vi "IrDA-Client.vi"() -> ()   [LabVIEW 2019]
doc: "Demonstrates how to open a connection to an IrDA server, read the data being sent, and display the data on a chart. This VI is designed to stop if the IrDA connection is terminated."
panel:
  in  "Server Closed":string="The server VI closed the connection."
  out "Waveform Graph":dbl[](graph)
  in  "Stop":bool
  # "Overview: Demonstrates the use of the IrDA functions to connect to an IrDA server VI and receive data.\nRequirements: IrDA-enabled computer\nInstructions:\n1. Ensure Simple IrDA - Server.vi is already running.\n2. Run the VI.\n3. Click Stop to stop the VI. Note that if you stop the server VI, this VI will stop automatically."
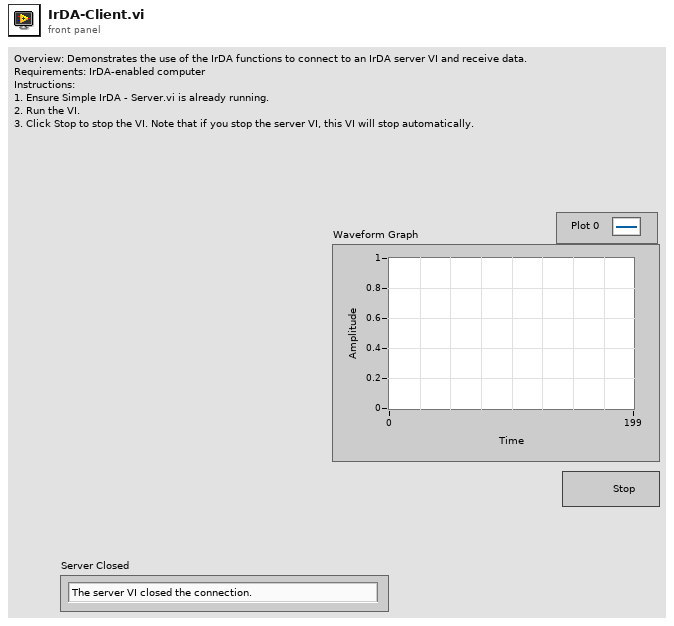
[diagram p1: front panel]
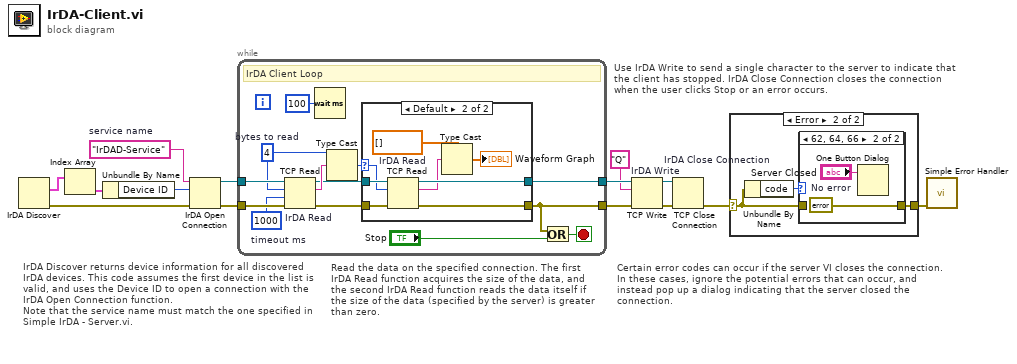
[diagram p0: block diagram]
diagram:
  w8 = "IrDAD-Service"  # service name
  # "Certain error codes can occur if the server VI closes the connection. In these cases, ignore the potential errors that can occur, and instead pop up a dialog indicating that the server closed the connection."
  # "Use IrDA Write to send a single character to the server to indicate that the client has stopped. IrDA Close Connection closes the connection when the user clicks Stop or an error occurs."
  # "Read the data on the specified connection. The first IrDA Read function acquires the size of the data, and the second IrDA Read function reads the data itself if the size of the data (specified by the server) is greater than zero."
  # "IrDA Discover returns device information for all discovered IrDA devices. This code assumes the first device in the list is valid, and uses the Device ID to open a connection with the IrDA Open Connection function. \nNote that the service name must match the one specified in Simple IrDA - Server.vi."
  n1 = IrDA Discover() -> (0:w10:errorcluster, 2:w12:cluster{"Device ID":u32, "Device Name":string}[])  [unwired: 1 in, 1 out]
  n2 = Index Array(array=w12) -> (element=w11:cluster{"Device ID":u32, "Device Name":string})  [unwired: 1 in]
  n3 = Unbundle By Name(w11) -> ("Device ID"=w9:u32)
  n4 = IrDA Open Connection(8:w10, 10:w9, 11:w8) -> (0:w13:errorcluster, 3:w14:refnum<k19>)  [unwired: 1 in]
  n5 = while {
    tunnel: w13 -> [w23]
    tunnel: w14 -> [w24]
    tunnel: [w19] -> w6
    tunnel: [w18] -> w4
    stop <- w21 stop-if-true
    w15 = 4  # bytes to read
    w16 = 1000  # timeout ms
    # "IrDA Client Loop"
    n6 = TCP Read "IrDA Read"(connection ID=w24, bytes to read=w15, error in (no error)=w23, 9:w16) -> (connection ID out=w26:refnum<k19>, data out=w27:string, error out=w25:errorcluster)  [unwired: 1 in]
    n7 = Wait (ms)(milliseconds to wait=u32 100) -> ()  [unwired: 1 out]
    n8 = Type Cast(type=w15, x=w27) -> (*(type *) &x=w17:i32)
    n9 = case shown="Default" w17 {
      selector: w17 -> [_ w30]
      tunnel: w26 -> [w29 w37]
      tunnel: w25 -> [w28 w36]
      tunnel: [w29 w33] -> w19
      tunnel: [w28 w32] -> w18
      frame ..0 {
        # "The server has not written any data"
      }
      frame Default {
        n10 = TCP Read "IrDA Read"(connection ID=w37, bytes to read=w30, error in (no error)=w36) -> (connection ID out=w33:refnum<k19>, data out=w31:string, error out=w32:errorcluster)  [unwired: 2 in]
        n11 = Type Cast(type=dbl[] [] ("chart"), x=w31) -> (*(type *) &x=→"Waveform Graph":dbl[])
      }
    }
    n12 = Or(x=w18, y="Stop") -> (x .or. y?=w21:bool)
  }
  n13 = TCP Write "IrDA Write"(connection ID=w6, data in="Q", error in (no error)=w4) -> (connection ID out=w7:refnum<k19>, error out=w5:errorcluster)  [unwired: 2 out]
  n14 = TCP Close Connection "IrDA Close Connection"(connection ID=w7, error in (no error)=w5) -> (error out=w2:errorcluster)  [unwired: 1 in, 1 out]
  n15 = case shown="Error" w2 {
    selector: w2 -> [w38 w40]
    tunnel: [w38 w39] -> w1
    frame No Error {
    }
    frame Error {
      n16 = Unbundle By Name(w40) -> ("code"=w41:i32)
      n17 = case shown="62, 64, 66" w41 {
        tunnel: w40 -> [w42 _]
        tunnel: [w42 w44] -> w39
        frame Default {
        }
        frame 62, 64, 66 {
          w44 = errorcluster {"status"=FALSE, "code"=0, "source"=""}  # No error
          n18 = One Button Dialog(message="Server Closed") -> ()  [unwired: 1 in, 1 out]
        }
      }
    }
  }
  n19 = call <vilib>:"Simple Error Handler.vi"("error in (no error)"=w1) -> ()  [unwired: 4 in, 5 out]
